vi "RSNRPZ Set Sensor Name.vi"(8 "error in (no error)":errorcluster, 9 "Name (\"\")":string, 10 "Channel (1)":i32=1, 11 "VISA session":refnum<visa-resource-name> caption="VISA resource name") -> (0 "error out":errorcluster, 3 "dup VISA session":refnum<visa-resource-name> caption="VISA resource name")   [LabVIEW 2010]
doc: "Sets a User Selected Sensor Name. This function is for the \"new\" sensor generation only (NRPxxS[N], NRPxxA[N], NRPxxT[N]).\nSets a name of the sensors according to the users requirements. The name specified by 'pName' will be displayed on the WebGUI of the network sensors. The sensor name given here is independent from the hostname of the sensor. However, if the sensor name is not yet specified it defaults to the hostname.\n\nRemote-control command(s):\nSYST:NAME"
uses:
  rsnrpz_32.dll
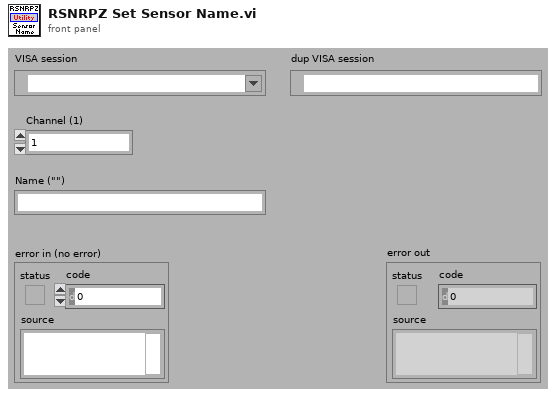
[diagram p1: front panel]
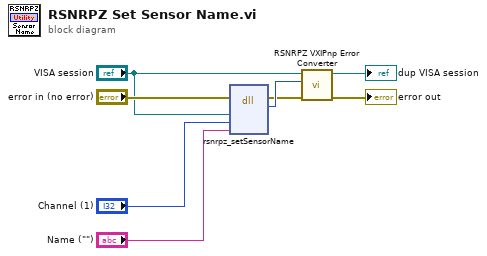
[diagram p0: block diagram]
diagram:
  n1 = dll-call lib="rsnrpz_32.dll" fn="rsnrpz_setSensorName"(error in="error in (no error)", "Instrument Handle"="VISA session", "Channel"="Channel (1)", "Name"="Name (\"\")") -> (error out=w5:errorcluster, w6:i32)  [unwired: 5 in, 1 out]
  n2 = call <instrlib>:"RSNRPZ VXIPnp Error Converter.vi"("error in"=w5, "VXIPnp error code"=w6, "VISA session"="VISA session") -> ("error out"=→"error out":errorcluster, "dup VISA session"=→"dup VISA session":refnum<visa-resource-name>)  [unwired: 7 in]
